vi "write_params.vi"(8 "error in (no error)":errorcluster, 10 "params":T1={"kernel"="rbf", "degree"=0.0, "gamma"={"gamma_type"="scale", "gamma_float"=0.001}, "coef0"=0.0, "tol"=0.001, "C"=1.0, "epsilon"=0.1, "shrinking"=TRUE, "cache_size"=200.0, "verbose"=FALSE, "max_iter"=-1.0}, 11 "SVR in":refnum<class "SVR.lvclass">) -> (0 "error out":errorcluster, 3 "SVR out":refnum<class "SVR.lvclass">)   [LabVIEW 2020, in "SVR.lvclass"]
uses:
  SVR.lvclass
  Controls/svr_params.ctl
  SVR.lvclass/SVR.ctl
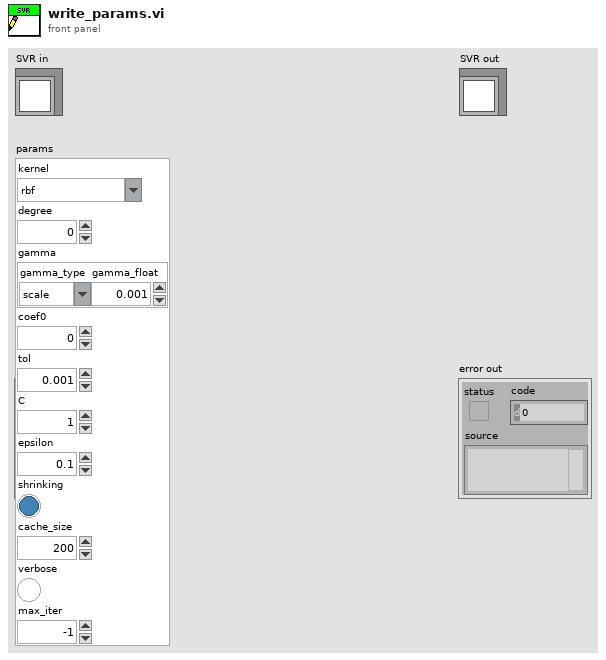
[diagram p1: front panel]
types:
  T1 = typedef "svr_params.ctl" = cluster{"kernel":string, "degree":dbl, "gamma":cluster{"gamma_type":string, "gamma_float":dbl}, "coef0":dbl, "tol":dbl, "C":dbl, "epsilon":dbl, "shrinking":bool, "cache_size":dbl, "verbose":bool, "max_iter":dbl}
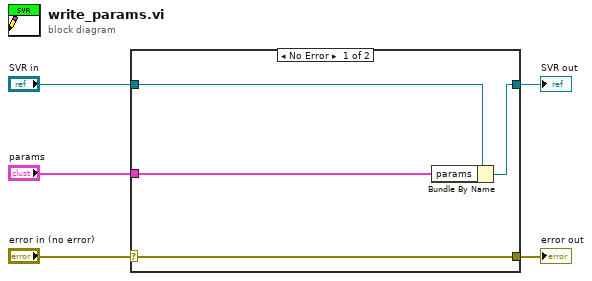
[diagram p0: block diagram]
diagram:
  n1 = case shown="No Error" "error in (no error)" {
    selector: "error in (no error)" -> [w9 w10]
    tunnel: [w9 w10] -> w4
    tunnel: [w7 w11] -> w2
    tunnel: "SVR in" -> [w8 w11]
    tunnel: "params" -> [w6 _]
    frame No Error {
      n2 = Bundle By Name(cluster=w8, "params"=w6) -> (w7:refnum<class "SVR.lvclass">)
    }
    frame Error {
    }
  }
  "error out" <- w4
  "SVR out" <- w2
